vi "PC_SVG_Single.vi"() -> ()   [LabVIEW 2021]
uses:
  Signal Voltage Generation/Typedefs/Signal Generation Settings.ctl
  Signal Voltage Generation/Typedefs/Generation Types.ctl
  Signal Voltage Generation/Typedefs/Single Tone Settings.ctl
  Signal Voltage Generation/Typedefs/Waveform Type.ctl
  Signal Voltage Generation/Typedefs/Tone Settings.ctl
  Signal Voltage Generation/Typedefs/Timing & Trigger Settings.ctl
  Signal Voltage Generation/Typedefs/Trigger Settings.ctl
  Signal Voltage Generation/Typedefs/Timing Settings.ctl
  Signal Voltage Generation/DAQ_Signal Voltage Generation.lvlib
panel:
  out "Generated Voltage Waveforms":waveform(dbl)[](graph)=[{"t0"=timestamp(0 s since 1904-01-01), "dt"=1e-05, "Y"=array[100000 elements]}]
  out "error out":errorcluster
  in  "Signal Generation Settings":T1={"Generation Type"=enum."Single Tone", "Generation Time (s)"=1.0, "Voltage Offset (v)"=2.5, "Single Tone Settings"={"Waveform Type"=enum."Square Wave", "Frequency (Hz)"=102.0, "Amplitude (V)"=2.5, "Duty Cycle (%)"=20.0}, "Multi Tone Settings"=[]} {"Voltage Offset (v)" format="%.2p"; "Generation Time (s)" format="%.2p"; "Multi Tone Settings"."Amplitude (V)" format="%#.2p"; "Multi Tone Settings"."Frequency (Hz)" format="%#.2p"; "Single Tone Settings"."Duty Cycle (%)" format="%#.2p"; "Single Tone Settings"."Amplitude (V)" format="%#.2p"; "Single Tone Settings"."Frequency (Hz)" format="%#.2p"}
  # "Frequency (Hz)"
  # "Amplitude (V)"
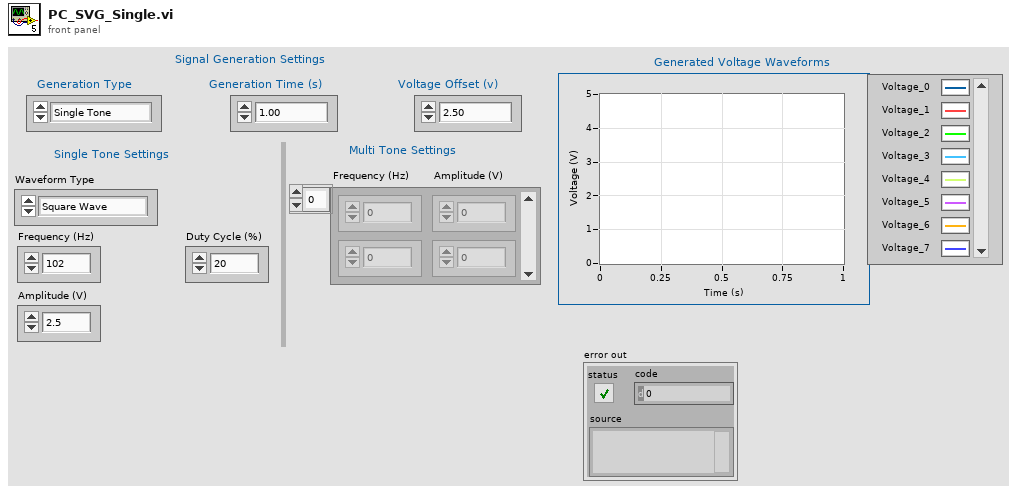
[diagram p1: front panel]
types:
  T1 = typedef "DAQ_Signal Voltage Generation.lvlib/Signal Generation Settings.ctl" = cluster{"Generation Type":T2, "Generation Time (s)":dbl, "Voltage Offset (v)":dbl, "Single Tone Settings":T3, "Multi Tone Settings":T5[]}
  T2 = typedef "DAQ_Signal Voltage Generation.lvlib/Generation Types.ctl" = enum16{"Single Tone", "Multi Tone"}
  T3 = typedef "DAQ_Signal Voltage Generation.lvlib/Single Tone Settings.ctl" = cluster{"Waveform Type":T4, "Frequency (Hz)":dbl, "Amplitude (V)":dbl, "Duty Cycle (%)":dbl}
  T4 = typedef "DAQ_Signal Voltage Generation.lvlib/Waveform Type.ctl" = enum16{"Sine Wave", "Square Wave"}
  T5 = typedef "DAQ_Signal Voltage Generation.lvlib/Tone Settings.ctl" = cluster{"Frequency (Hz)":dbl, "Amplitude (V)":dbl}
  T6 = typedef "DAQ_Signal Voltage Generation.lvlib/Timing & Trigger Settings.ctl" = cluster{"Trigger Settings":T7, "Timing Settings":T8}
  T7 = typedef "DAQ_Signal Voltage Generation.lvlib/Trigger Settings.ctl" = cluster{"Trigger Type":enum16{"No Trigger", "Digital Start"}, "Digital Start Trigger Source":tag, "Digital Start Trigger Edge":i32}
  T8 = typedef "DAQ_Signal Voltage Generation.lvlib/Timing Settings.ctl" = cluster{"Sample Clock Source":tag, "Sample Rate (Hz)":dbl}
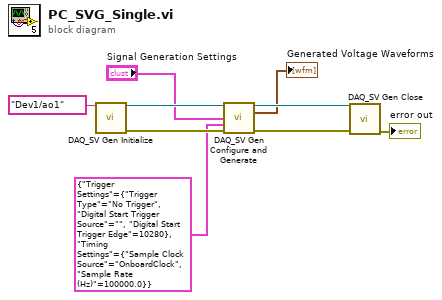
[diagram p0: block diagram]
diagram:
  n1 = call "DAQ_SV Gen Initialize.vi"("Physical Channels"=tag "Dev1/ao1") -> ("DAQmx Task Out"=w9:refnum<k21>, "error out"=w8:errorcluster)  [unwired: 13 in]
  n2 = call "DAQ_SV Gen Configure and Generate.vi"("DAQmx Task In"=w9, "Signal Generation Settings"="Signal Generation Settings", "Timing & Trigger Settings"=T6 {"Trigger Settings"={"Trigger Type"=enum."No Trigger", "Digital Start Trigger Source"="", "Digital Start Trigger Edge"=10280}, "Timing Settings"={"Sample Clock Source"="OnboardClock", "Sample Rate (Hz)"=100000.0}}, "error in"=w8) -> ("DAQmx Task Out"=w7:refnum<k21>, "Generated Voltage Waveforms"=→"Generated Voltage Waveforms":waveform(dbl)[], "error out"=w6:errorcluster)  [unwired: 9 in]
  n3 = call "DAQ_SV Gen Close.vi"("DAQmx Task In"=w7, "error in"=w6) -> ("error out"=→"error out":errorcluster)  [unwired: 13 in]
